vi "quiz1_punto_dentro_Poligono.vi"() -> ()   [LabVIEW 2018]
uses:
  <vilib>/Analysis/Matrix/Numeric/Conversions/Matrix To Array - RM.vi
  <vilib>/Analysis/Matrix/NI_Matrix.lvlib
panel:
  out "Punto dentro del Poligono":bool
  out "poligono":dbl[][](array[numeric]) format="%_4f"
  out "y":dbl
  out "x":dbl
  out "j":dbl
  in  "PosY":dbl[](array[numeric])=[6.5] caption="Y" format="%_4f"
  in  "PosX":dbl[](array[numeric])=[-65.5] caption="X" format="%_4f"
  out "XY Graph":cluster{"Array":dbl[], "Array 2":dbl[]}[](graph)
  in  "Latitud - VectorY":dbl[](array[numeric])=[5.5, 6.9, 4.8, 6.1, 3.6, 5.8, 5.5] format="%_4f"
  in  "Longitud - VectorX":dbl[](array[numeric])=[-68.3, -65.5, -61.9, -64.8, -64.9, -65.8, -68.3] format="%_4f"
  # "Latitud\nLa latitud proporciona la localización de \nun lugar, en dirección Norte o Sur desde \nel ecuador"
  # "Longitud\nLa longitud proporciona la localización \nde un lugar, en dirección Este u Oeste"
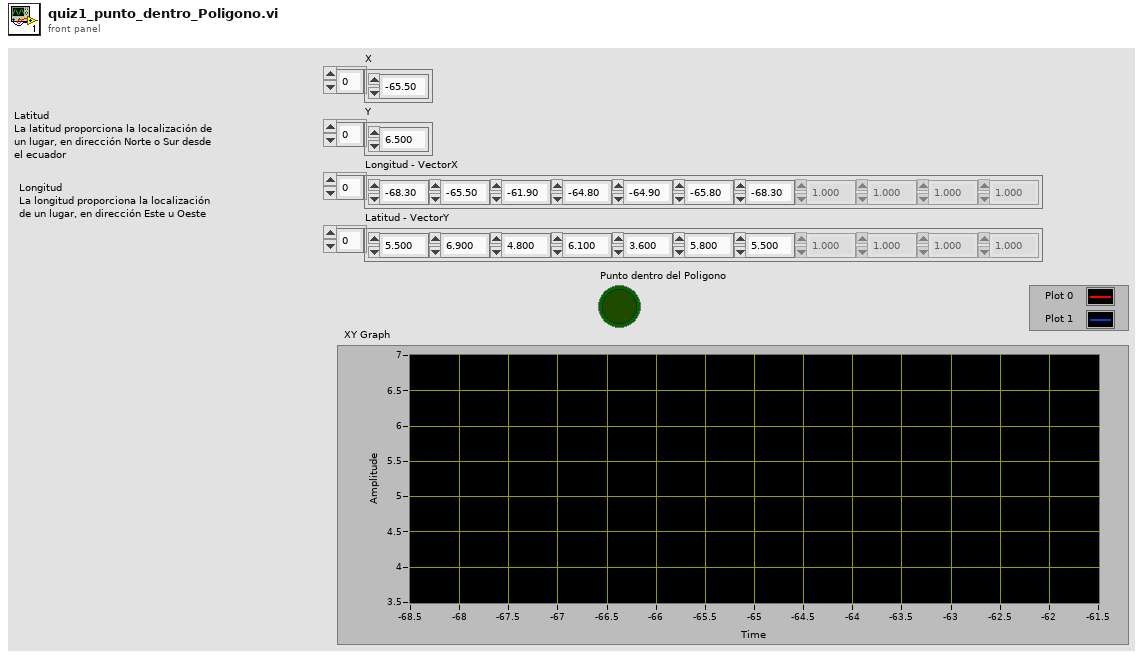
[diagram p1: front panel]
types:
  T1 = cluster{"Longitud - VectorX":dbl[], "Latitud - VectorY":dbl[]}
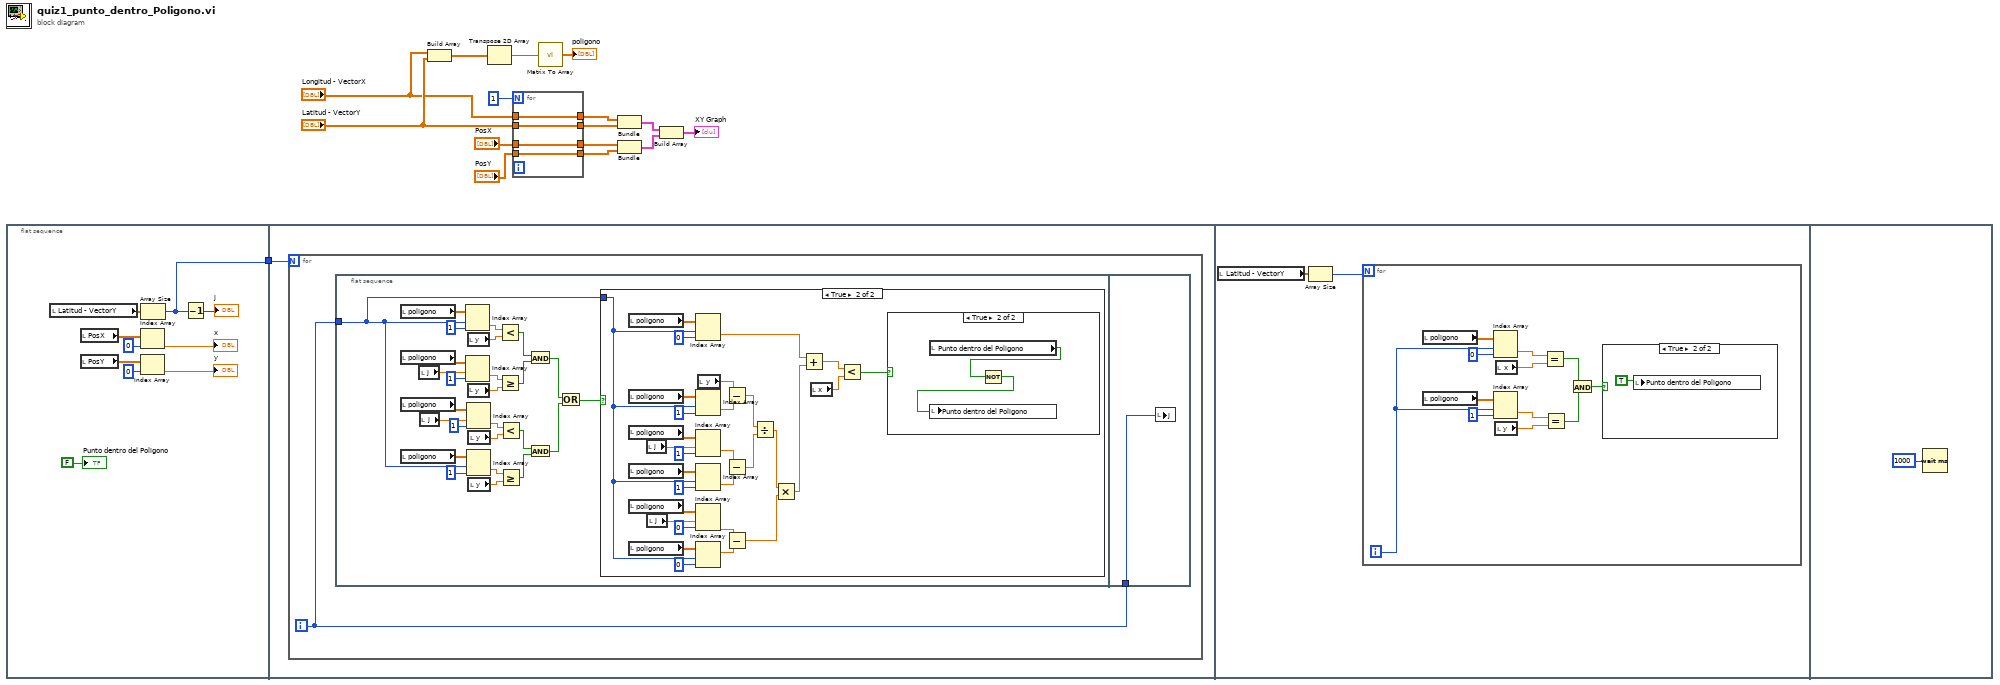
[diagram p0: block diagram]
diagram:
  n1 = flat-sequence {
    tunnel: [w18] -> w6
    tunnel: w6 -> [w27]
    frame #0 {
      n2 = local read "Latitud - VectorY"() -> (w20:dbl[])
      n3 = local read "PosX"() -> (w23:dbl[])
      n4 = local read "PosY"() -> (w26:dbl[])
      n5 = Index Array(array=w23, index=0) -> (element=→"x":dbl)
      n6 = Index Array(array=w26, index=0) -> (element=→"y":dbl)
      n7 = Array Size(array=w20) -> (size(s)=w18:i32)
      n8 = Decrement(x=w18) -> (x-1=→"j":i32)
      "Punto dentro del Poligono" <- FALSE ("punto")
    }
    frame #1 {
      n9 = for {
        N: w27 -> [_]
        i -> [w28]
        n10 = flat-sequence {
          tunnel: w28 -> [w29]
          tunnel: w28 -> [w87]
          frame #0 {
            n11 = local read "poligono"() -> (w54:dbl[][])
            n12 = local read "poligono"() -> (w47:dbl[][])
            n13 = local read "poligono"() -> (w42:dbl[][])
            n14 = local read "poligono"() -> (w35:dbl[][])
            n15 = local read "j"() -> (w46:dbl)
            n16 = local read "j"() -> (w43:dbl)
            n17 = Index Array(array=w54, index (row)=w29, index (col)=1 ("disabled index (col)")) -> (element=w52:dbl)
            n18 = Index Array(array=w47, index (row)=w46, index (col)=1 ("disabled index (col)")) -> (element=w49:dbl)
            n19 = Index Array(array=w42, index (row)=w43, index (col)=1 ("disabled index (col)")) -> (element=w40:dbl)
            n20 = Index Array(array=w35, index (row)=w29, index (col)=1 ("disabled index (col)")) -> (element=w37:dbl)
            n21 = local read "y"() -> (w51:dbl)
            n22 = local read "y"() -> (w50:dbl)
            n23 = local read "y"() -> (w39:dbl)
            n24 = local read "y"() -> (w38:dbl)
            n25 = Less?(x=w52, y=w51) -> (x < y?=w44:bool)
            n26 = Greater Or Equal?(x=w49, y=w50) -> (x >= y?=w45:bool)
            n27 = Less?(x=w40, y=w39) -> (x < y?=w34:bool)
            n28 = Greater Or Equal?(x=w37, y=w38) -> (x >= y?=w33:bool)
            n29 = And(x=w44, y=w45) -> (x .and. y?=w32:bool)
            n30 = And(x=w34, y=w33) -> (x .and. y?=w31:bool)
            n31 = Or(x=w32, y=w31) -> (x .or. y?=w30:bool)
            n32 = case shown="True" w30 {
              tunnel: w29 -> [_ w65]
              frame False {
              }
              frame True {
                n33 = local read "poligono"() -> (w83:dbl[][])
                n34 = local read "poligono"() -> (w81:dbl[][])
                n35 = local read "poligono"() -> (w76:dbl[][])
                n36 = local read "poligono"() -> (w73:dbl[][])
                n37 = local read "poligono"() -> (w69:dbl[][])
                n38 = local read "poligono"() -> (w67:dbl[][])
                n39 = local read "j"() -> (w75:dbl)
                n40 = local read "j"() -> (w70:dbl)
                n41 = Index Array(array=w83, index (row)=w65, index (col)=0 ("disabled index (col)")) -> (element=w82:dbl)
                n42 = Index Array(array=w81, index (row)=w65, index (col)=1 ("disabled index (col)")) -> (element=w78:dbl)
                n43 = Index Array(array=w76, index (row)=w75, index (col)=1 ("disabled index (col)")) -> (element=w71:dbl)
                n44 = Index Array(array=w73, index (row)=w65, index (col)=1 ("disabled index (col)")) -> (element=w72:dbl)
                n45 = Index Array(array=w69, index (row)=w70, index (col)=0 ("disabled index (col)")) -> (element=w63:dbl)
                n46 = Index Array(array=w67, index (row)=w65, index (col)=0 ("disabled index (col)")) -> (element=w64:dbl)
                n47 = local read "y"() -> (w79:dbl)
                n48 = Subtract(x=w79, y=w78) -> (x-y=w62:dbl)
                n49 = Subtract(x=w71, y=w72) -> (x-y=w61:dbl)
                n50 = Subtract(x=w63, y=w64) -> (x-y=w60:dbl)
                n51 = Divide(x=w62, y=w61) -> (x/y=w59:dbl)
                n52 = Multiply(x=w59, y=w60) -> (x*y=w58:dbl)
                n53 = Add(x=w82, y=w58) -> (x+y=w57:dbl)
                n54 = local read "x"() -> (w56:dbl)
                n55 = Less?(x=w57, y=w56) -> (x < y?=w55:bool)
                n56 = case shown="True" w55 {
                  frame False {
                  }
                  frame True {
                    n57 = local read "Punto dentro del Poligono"() -> (w86:bool)
                    n58 = Not(x=w86) -> (.not. x?=w85:bool)
                    n59 = local write "Punto dentro del Poligono"(w85) -> ()
                  }
                }
              }
            }
          }
          frame #1 {
            n60 = local write "j"(w87) -> ()
          }
        }
      }
    }
    frame #2 {
      n61 = local read "Latitud - VectorY"() -> (w89:dbl[])
      n62 = Array Size(array=w89) -> (size(s)=w88:i32)
      n63 = for {
        N: w88 -> [_]
        i -> [w97]
        n64 = local read "poligono"() -> (w101:dbl[][])
        n65 = local read "poligono"() -> (w98:dbl[][])
        n66 = Index Array(array=w101, index (row)=w97, index (col)=0 ("disabled index (col)")) -> (element=w95:dbl)
        n67 = Index Array(array=w98, index (row)=w97, index (col)=1 ("disabled index (col)")) -> (element=w94:dbl)
        n68 = local read "y"() -> (w93:dbl)
        n69 = local read "x"() -> (w96:dbl)
        n70 = Equal?(x=w95, y=w96) -> (x = y?=w92:bool)
        n71 = Equal?(x=w94, y=w93) -> (x = y?=w91:bool)
        n72 = And(x=w92, y=w91) -> (x .and. y?=w90:bool)
        n73 = case shown="True" w90 {
          frame False {
          }
          frame True {
            n74 = local write "Punto dentro del Poligono"(TRUE) -> ()
          }
        }
      }
    }
    frame #3 {
      n75 = Wait (ms)(milliseconds to wait=u32 1000) -> ()  [unwired: 1 out]
    }
  }
  n76 = Build Array("Longitud - VectorX", "Latitud - VectorY") -> (w1:dbl[][])
  n77 = Transpose 2D Array(2D array=w1) -> (transposed array=w5:dbl[][])
  n78 = for {
    N: 1 -> [_]
    tunnel: [w107] -> w15
    tunnel: [w106] -> w14
    tunnel: [w105] -> w13
    tunnel: [w104] -> w12
    tunnel: "Longitud - VectorX" -> [w107]
    tunnel: "Latitud - VectorY" -> [w106]
    tunnel: "PosX" -> [w105]
    tunnel: "PosY" -> [w104]
  }
  n79 = call-poly <vilib>:"Matrix To Array.vi"("Real Matrix"=w5) -> ("Real 2D Array"=→"poligono":dbl[][])
  n80 = Bundle("Longitud - VectorX"=w15, "Latitud - VectorY"=w14) -> (w11:T1)  [unwired: 1 in]
  n81 = Bundle("PosX"=w13, "PosY"=w12) -> (w10:cluster{"PosX":dbl[], "PosY":dbl[]})  [unwired: 1 in]
  n82 = Build Array(w11, w10) -> (→"XY Graph":cluster{"PosX":dbl[], "PosY":dbl[]}[])
